vi "Conv_JSON_2 (SubVI).vi"(9 "data":cluster{"name":string}={"name"="i_range"}, 11 "Cluster":T1) -> (3 "String":string)   [LabVIEW 2015]
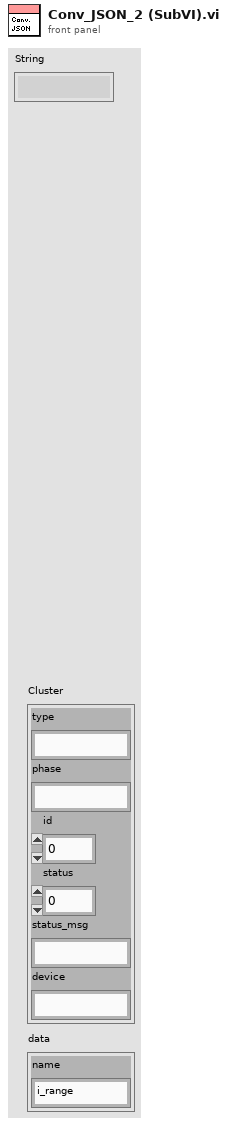
[diagram p1: front panel]
types:
  T1 = cluster{"type":string, "phase":string, "id":u8, "status":i32, "status_msg":string, "device":string}
  T2 = cluster{"type":string, "phase":string, "id":u8, "status":i32, "status_msg":string, "device":string, "data":cluster{"name":string}}
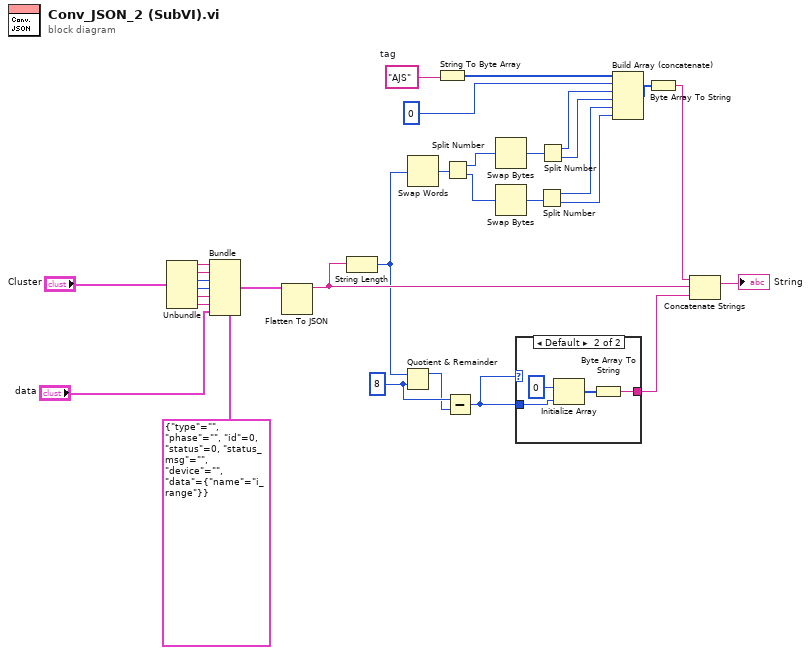
[diagram p0: block diagram]
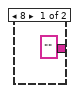
[diagram p2: hidden frame]
diagram:
  w5 = 8 ("y")
  w26 = "AJS"  # tag
  n1 = Unbundle("Cluster") -> ("type"=w15:string, "phase"=w14:string, "id"=w13:u8, "status"=w12:i32, "status_msg"=w11:string, "device"=w10:string)
  n2 = Bundle(cluster=T2 {"type"="", "phase"="", "id"=0, "status"=0, "status_msg"="", "device"="", "data"={"name"="i_range"}}, "type"=w15, "phase"=w14, "id"=w13, "status"=w12, "status_msg"=w11, "device"=w10, "data"="data") -> (w8:T2)
  n3 = Flatten To JSON(anything=w8) -> (JSON string=w30:string)  [unwired: 2 in, 1 out]
  n4 = String Length(string=w30) -> (length=w2:i32)
  n5 = Quotient & Remainder(x=w2, y=w5) -> (x-y*floor(x/y)=w4:i32)  [unwired: 1 out]
  n6 = Swap Words(1:w2) -> (0:w29:i32)
  n7 = String To Byte Array(string=w26) -> (unsigned byte array=w25:u8[])
  n8 = Split Number(x=w29) -> (hi(x)=w28:u16, lo(x)=w27:u16)
  n9 = Subtract(x=w5, y=w4) -> (x-y=w3:i32)
  n10 = Swap Bytes(anything=w28) -> (byte swapped=w20:u16)
  n11 = Swap Bytes(anything=w27) -> (byte swapped=w21:u16)
  n12 = case shown="Default" w3 {
    tunnel: ["" ("string") w34] -> w1
    tunnel: w3 -> [_ w33]
    frame 8 {
    }
    frame Default {
      n13 = Initialize Array(u8 0 ("element"), w33) -> (w35:u8[])
      n14 = Byte Array To String(unsigned byte array=w35) -> (string=w34:string)
    }
  }
  n15 = Split Number(x=w21) -> (hi(x)=w17:u8, lo(x)=w16:u8)
  n16 = Split Number(x=w20) -> (hi(x)=w19:u8, lo(x)=w18:u8)
  n17 = Build Array (concatenate)(w25, u8 0, w19, w18, w17, w16) -> (w23:u8[])
  n18 = Byte Array To String(unsigned byte array=w23) -> (string=w22:string)
  n19 = Concatenate Strings(w22, w30, w1) -> (→"String":string)
